vi "Auto 7.vi"(8 "Error In":errorcluster) -> (0 "Error Out":errorcluster)   [LabVIEW 2014]
uses:
  Global Variables/Refnum Names.vi
  <vilib>/Rock Robotics/Network Tables/SD Read Boolean.vi
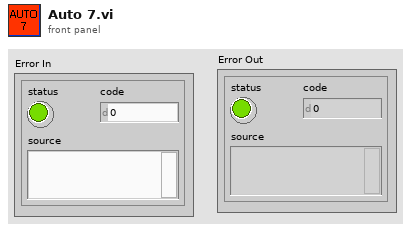
[diagram p1: front panel]
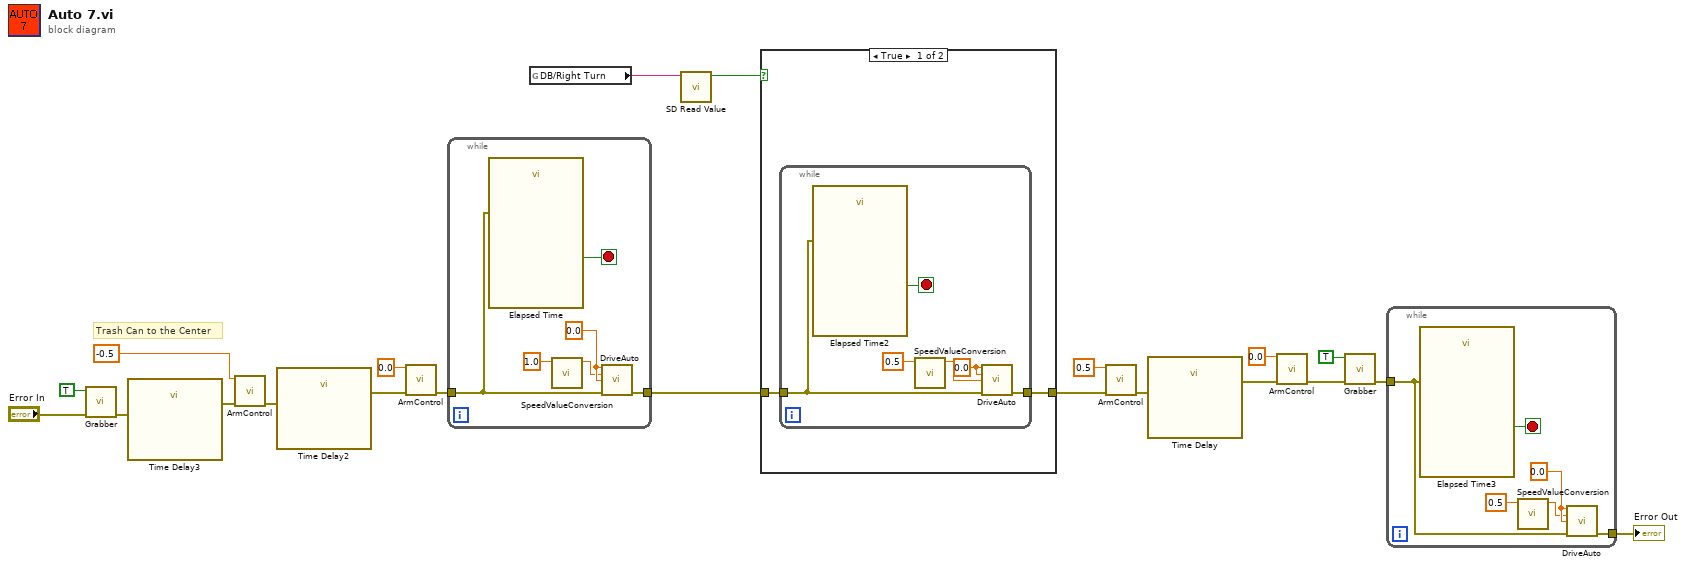
[diagram p0: block diagram]
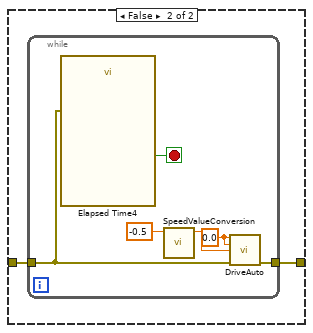
[diagram p2: hidden frame]
diagram:
  # "Trash Can to the Center"
  n1 = call "Grabber.vi"("Error In"="Error In", "Grabber Open/Close"=TRUE) -> ("Error Out"=w9:errorcluster)  [unwired: 9 in]
  n2 = call "Time Delay3"("error in (no error)"=w9) -> ("error out"=w16:errorcluster)  [unwired: 10 in]
  n3 = call "ArmControl.vi"("Arm Value"=-0.5, "Error In"=w16) -> ("Error Out"=w21:errorcluster)  [unwired: 13 in]
  n4 = call "Time Delay2"("error in (no error)"=w21) -> ("error out"=w18:errorcluster)  [unwired: 10 in]
  n5 = call "ArmControl.vi"("Arm Value"=0.0, "Error In"=w18) -> ("Error Out"=w15:errorcluster)  [unwired: 13 in]
  n6 = while {
    tunnel: w15 -> [w24]
    tunnel: [w27] -> w12
    stop <- w25 stop-if-true
    w26 = 0.0 ("Arm Value")
    n7 = call "Elapsed Time"("error in (no error)"=w24) -> ("Time has Elapsed"=w25:bool)  [unwired: 11 in, 7 out]
    n8 = call "SpeedValueConversion.vi"("Motor Value In"=1.0 ("X In")) -> ("New to Old Conversion Value Out"=w22:dbl)  [unwired: 9 in, 1 out]
    n9 = call "DriveAuto.vi"("X In"=w26, "Y In"=w22, "R In"=w26, "Error In"=w24) -> ("Error Out"=w27:errorcluster)  [unwired: 11 in]
  }
  n10 = global read "Refnum Names.vi" "DB/Right Turn"() -> (w1:string)
  n11 = call-poly <vilib>:"SD Read Value.vi"("Name"=w1) -> ("Boolean"=w14:bool)  [unwired: 8 in, 2 out]
  n12 = case shown="True" w14 {
    tunnel: w12 -> [w29 w37]
    tunnel: [w28 w36] -> w13
    frame True {
      n13 = while {
        tunnel: w29 -> [w32]
        tunnel: [w35] -> w28
        stop <- w33 stop-if-true
        w34 = 0.0 ("Arm Value")
        n14 = call "Elapsed Time2"("error in (no error)"=w32) -> ("Time has Elapsed"=w33:bool)  [unwired: 11 in, 7 out]
        n15 = call "SpeedValueConversion.vi"("Motor Value In"=0.5 ("X In")) -> ("New to Old Conversion Value Out"=w30:dbl)  [unwired: 9 in, 1 out]
        n16 = call "DriveAuto.vi"("X In"=w34, "Y In"=w34, "R In"=w30, "Error In"=w32) -> ("Error Out"=w35:errorcluster)  [unwired: 11 in]
      }
    }
    frame False {
      n17 = while {
        tunnel: w37 -> [w40]
        tunnel: [w42] -> w36
        stop <- w41 stop-if-true
        w43 = 0.0 ("Arm Value")
        n18 = call "Elapsed Time4"("error in (no error)"=w40) -> ("Time has Elapsed"=w41:bool)  [unwired: 11 in, 7 out]
        n19 = call "SpeedValueConversion.vi"("Motor Value In"=-0.5 ("X In")) -> ("New to Old Conversion Value Out"=w38:dbl)  [unwired: 9 in, 1 out]
        n20 = call "DriveAuto.vi"("X In"=w43, "Y In"=w43, "R In"=w38, "Error In"=w40) -> ("Error Out"=w42:errorcluster)  [unwired: 11 in]
      }
    }
  }
  n21 = call "ArmControl.vi"("Arm Value"=0.5, "Error In"=w13) -> ("Error Out"=w19:errorcluster)  [unwired: 13 in]
  n22 = call "Time Delay"("error in (no error)"=w19) -> ("error out"=w17:errorcluster)  [unwired: 10 in]
  n23 = call "ArmControl.vi"("Arm Value"=0.0, "Error In"=w17) -> ("Error Out"=w3:errorcluster)  [unwired: 13 in]
  n24 = call "Grabber.vi"("Error In"=w3, "Grabber Open/Close"=TRUE) -> ("Error Out"=w2:errorcluster)  [unwired: 9 in]
  n25 = while {
    tunnel: w2 -> [w46]
    tunnel: [w49] -> w20
    stop <- w47 stop-if-true
    w48 = 0.0 ("Arm Value")
    n26 = call "Elapsed Time3"("error in (no error)"=w46) -> ("Time has Elapsed"=w47:bool)  [unwired: 11 in, 7 out]
    n27 = call "SpeedValueConversion.vi"("Motor Value In"=0.5 ("X In")) -> ("New to Old Conversion Value Out"=w44:dbl)  [unwired: 9 in, 1 out]
    n28 = call "DriveAuto.vi"("X In"=w48, "Y In"=w44, "R In"=w48, "Error In"=w46) -> ("Error Out"=w49:errorcluster)  [unwired: 11 in]
  }
  "Error Out" <- w20
